vi "Update system definition tree from fom info.vi"(8 "error in":errorcluster, 9 "Interactions":T1[](array[typedef]), 10 "Objects":T2[](array[typedef]), 11 "Item Ref in":T3 format="%.0x") -> (0 "error out":errorcluster, 3 "Item Ref out":T3 format="%.0x")   [LabVIEW 2019, in "HLA Custom Device System Explorer.lvlib"]
uses:
  HLA Custom Device System Explorer.lvlib
  <vilib>/NI VeriStand/Custom Device API/Custom Device Item Ref.ctl
  FOM/_typedefs/object_instance_json_type.ctl
  FOM/_typedefs/interaction_json_type.ctl
  Shared/Constants.vi
  <vilib>/NI VeriStand/Custom Device API/Custom Device API.lvlib
  Shared/HLA Custom Device Shared.lvlib
  <vilib>/Utility/SystemLogging/NI_SystemLogging.lvlib
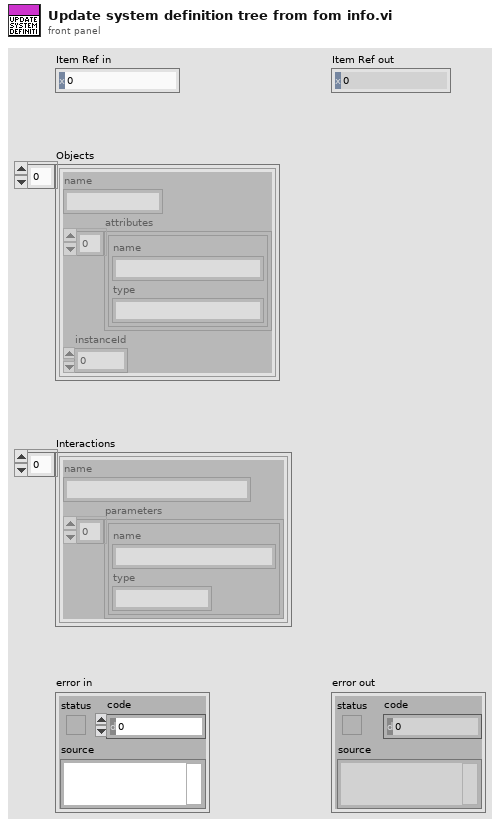
[diagram p1: front panel]
types:
  T1 = typedef "HLA Custom Device System Explorer.lvlib/interaction_json_type.ctl" = cluster{"name":string, "parameters":cluster{"name":string, "type":string}[]}
  T2 = typedef "HLA Custom Device System Explorer.lvlib/object_instance_json_type.ctl" = cluster{"name":string, "attributes":cluster{"name":string, "type":string}[], "instanceId":i32}
  T3 = typedef "Custom Device API.lvlib/Custom Device Item Ref.ctl" = u64
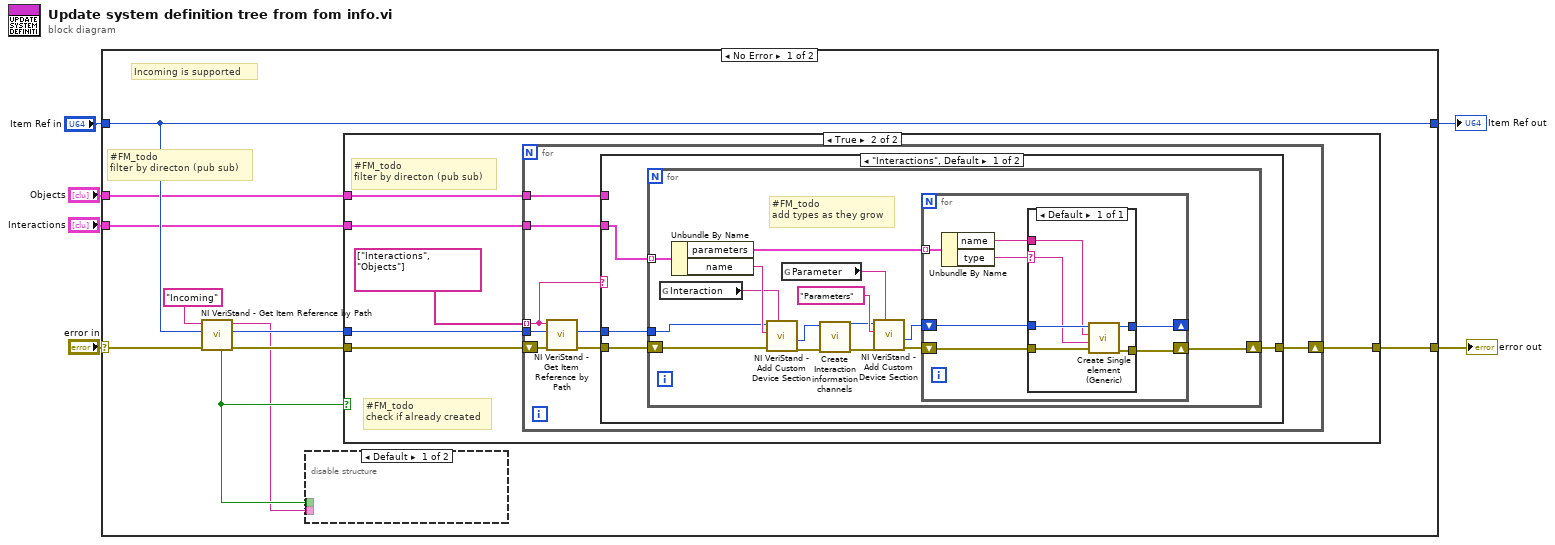
[diagram p0: block diagram]
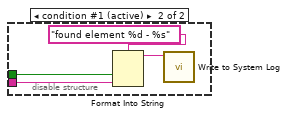
[diagram p2: hidden frame]
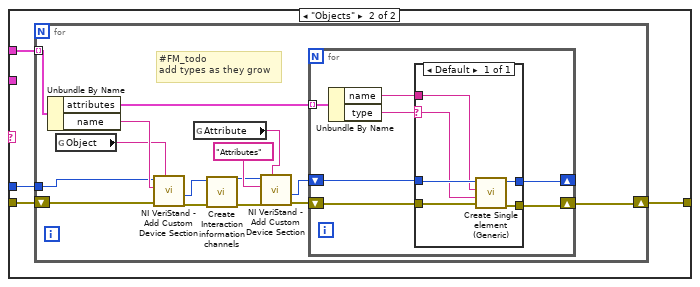
[diagram p4: hidden frame]
diagram:
  n1 = case shown="No Error" "error in" {
    selector: "error in" -> [w14 w100]
    tunnel: [w10 w100] -> w5
    tunnel: [w15 w101] -> w4
    tunnel: "Item Ref in" -> [w15 w101]
    tunnel: "Objects" -> [w12 _]
    tunnel: "Interactions" -> [w11 _]
    frame No Error {
      # "#FM_todo\nfilter by directon (pub sub)"
      # "Incoming is supported"
      n2 = call <vilib>:"NI VeriStand - Get Item Reference by Path.vi"("error in (no error)"=w14, "Root Ref"=w15, "Item Path in"="Incoming") -> ("error out"=w9:errorcluster, "Item Ref"=w13:T3, "Item Path out"=w7:string, "Found"=w8:bool)  [unwired: 5 in]
      n3 = disable-structure shown="Default" {
        disable-tunnel: w8 -> [_ w18]
        disable-tunnel: w7 -> [_ w19]
        frame condition #0 {
        }
        frame condition #1 (active) {
          n4 = Format Into String(format string="found element %d - %s", w18, w19) -> (resulting string=w20:string)  [unwired: 2 in, 1 out]
          n5 = call <vilib>:"Write to System Log.vi"("message"=w20) -> ()  [unwired: 10 in, 1 out]
        }
      }
      n6 = case shown="True" w8 {
        tunnel: w13 -> [_ w26]
        tunnel: w12 -> [_ w23]
        tunnel: w11 -> [_ w24]
        tunnel: w9 -> [w21 w27]
        tunnel: [w21 w22] -> w10
        frame False {
        }
        frame True {
          # "#FM_todo\ncheck if already created"
          # "#FM_todo\nfilter by directon (pub sub)"
          n7 = for {
            tunnel: w26 -> [w34]
            tunnel: string[] ["Interactions", "Objects"] ("Item Path in") -> [w29] mode=indexing
            tunnel: w24 -> [w31]
            tunnel: w23 -> [w28]
            shift-right: [w30] -> w22
            shift-left: w27 -> [w35]
            n8 = call <vilib>:"NI VeriStand - Get Item Reference by Path.vi"("error in (no error)"=w35, "Root Ref"=w34, "Item Path in"=w29) -> ("error out"=w32:errorcluster, "Item Ref"=w33:T3)  [unwired: 5 in, 2 out]
            n9 = case shown="\"Interactions\", Default" w29 {
              tunnel: w33 -> [w39 w71]
              tunnel: w32 -> [w38 w70]
              tunnel: w31 -> [w36 _]
              tunnel: [w37 w69] -> w30
              tunnel: w28 -> [_ w68]
              frame "Interactions", Default {
                n10 = for {
                  shift-right: [w51] -> w37
                  shift-left: w38 -> [w53]
                  tunnel: w39 -> [w52]
                  tunnel: w36 -> [w42] mode=indexing
                  # "#FM_todo\nadd types as they grow"
                  n11 = global read "Constants.vi" "Interaction"() -> (w40:string)
                  n12 = Unbundle By Name(w42) -> ("parameters"=w50:cluster{"name":string, "type":string}[], "name"=w54:string)
                  n13 = call <vilib>:"NI VeriStand - Add Custom Device Section.vi"("GUID (Default Section)"=w40, "error in (no error)"=w53, "Section Name"=w54, "Parent Ref in"=w52) -> ("error out"=w48:errorcluster, "Section Ptr"=w49:T3)  [unwired: 4 in, 2 out]
                  n14 = global read "Constants.vi" "Parameter"() -> (w41:string)
                  n15 = call "Create Interaction information channels.vi"("error in"=w48, "Item Ref in"=w49) -> ("error out"=w46:errorcluster, "Item Ref out"=w45:T3)  [unwired: 8 in]
                  n16 = call <vilib>:"NI VeriStand - Add Custom Device Section.vi"("GUID (Default Section)"=w41, "error in (no error)"=w46, "Section Name"="Parameters", "Parent Ref in"=w45) -> ("error out"=w43:errorcluster, "Section Ptr"=w44:T3)  [unwired: 4 in, 2 out]
                  n17 = for {
                    shift-right: [w57] -> w51
                    shift-left: w43 -> [w61]
                    tunnel: w50 -> [w56] mode=indexing
                    shift-right: [w58] -> _
                    shift-left: w44 -> [w60]
                    n18 = Unbundle By Name(w56) -> ("name"=w59:string, "type"=w55:string)
                    n19 = case shown="Default" w55 {
                      selector: w55 -> [w65]
                      tunnel: w61 -> [w66]
                      tunnel: w60 -> [w67]
                      tunnel: w59 -> [w62]
                      tunnel: [w64] -> w58
                      tunnel: [w63] -> w57
                      frame Default {
                        n20 = call "Create Single element (Generic).vi"("error in"=w66, "type"=w65, "name"=w62, "Item Ref in"=w67) -> ("error out"=w63:errorcluster, "Item Ref out"=w64:T3)  [unwired: 6 in]
                      }
                    }
                  }
                }
              }
              frame "Objects" {
                n21 = for {
                  shift-right: [w83] -> w69
                  shift-left: w70 -> [w85]
                  tunnel: w68 -> [w80] mode=indexing
                  tunnel: w71 -> [w84]
                  # "#FM_todo\nadd types as they grow"
                  n22 = Unbundle By Name(w80) -> ("attributes"=w82:cluster{"name":string, "type":string}[], "name"=w86:string)
                  n23 = global read "Constants.vi" "Object"() -> (w81:string)
                  n24 = call <vilib>:"NI VeriStand - Add Custom Device Section.vi"("GUID (Default Section)"=w81, "error in (no error)"=w85, "Section Name"=w86, "Parent Ref in"=w84) -> ("error out"=w78:errorcluster, "Section Ptr"=w79:T3)  [unwired: 4 in, 2 out]
                  n25 = global read "Constants.vi" "Attribute"() -> (w72:string)
                  n26 = call "Create Interaction information channels.vi"("error in"=w78, "Item Ref in"=w79) -> ("error out"=w76:errorcluster, "Item Ref out"=w75:T3)  [unwired: 8 in]
                  n27 = call <vilib>:"NI VeriStand - Add Custom Device Section.vi"("GUID (Default Section)"=w72, "error in (no error)"=w76, "Section Name"="Attributes", "Parent Ref in"=w75) -> ("error out"=w73:errorcluster, "Section Ptr"=w74:T3)  [unwired: 4 in, 2 out]
                  n28 = for {
                    shift-right: [w87] -> w83
                    shift-left: w73 -> [w91]
                    tunnel: w82 -> [w93] mode=indexing
                    shift-right: [w88] -> _
                    shift-left: w74 -> [w90]
                    n29 = Unbundle By Name(w93) -> ("name"=w89:string, "type"=w92:string)
                    n30 = case shown="Default" w92 {
                      selector: w92 -> [w96]
                      tunnel: w91 -> [w98]
                      tunnel: w90 -> [w99]
                      tunnel: w89 -> [w97]
                      tunnel: [w95] -> w88
                      tunnel: [w94] -> w87
                      frame Default {
                        n31 = call "Create Single element (Generic).vi"("error in"=w98, "type"=w96, "name"=w97, "Item Ref in"=w99) -> ("error out"=w94:errorcluster, "Item Ref out"=w95:T3)  [unwired: 6 in]
                      }
                    }
                  }
                }
              }
            }
          }
        }
      }
    }
    frame Error {
    }
  }
  "error out" <- w5
  "Item Ref out" <- w4
